vi "PalmSense Configure.vi"(8 "error in (no error)":errorcluster, 10 "Message Data":variant, 11 "Data Cluster":T1) -> (0 "error out":errorcluster, 2 "Send Resp":bool, 3 "Data Cluster out":T1)   [LabVIEW 2020, in "PalmSens.lvlib"]
uses:
  PalmSens.lvlib
  PalmSense Hardware Configuration.ctl
  <instrlib>/PalmSens SDK for LabVIEW 5.10/PalmSens/PalmSens.lvclass
  support/Message Queue/Message Cluster.ctl
  support/Message Queue/Message Queue.lvlib
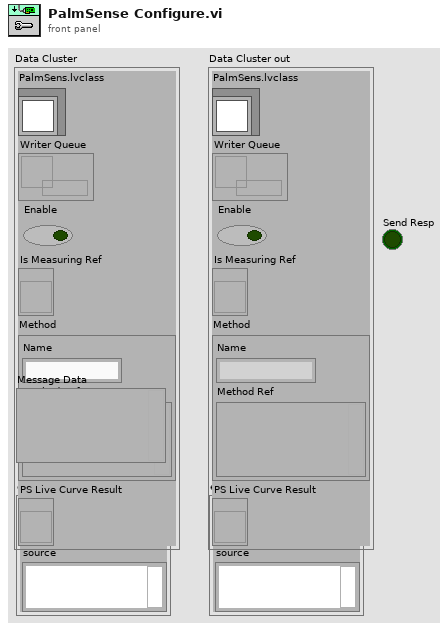
[diagram p1: front panel]
types:
  T1 = typedef "PalmSens.lvlib/PalmSense Hardware Configuration.ctl" = cluster{"PalmSens.lvclass":refnum<class "PalmSens.lvclass">, "Writer Queue":refnum<queue>, "Enable":bool, "Is Measuring Ref":refnum<vi>, "Method":cluster{"Name":string, "Method Ref":variant}, "PS Live Curve Result":refnum<vi>}
  T2 = typedef "Message Queue.lvlib/Message Cluster.ctl" = cluster{"Message":string, "Message Data":variant}
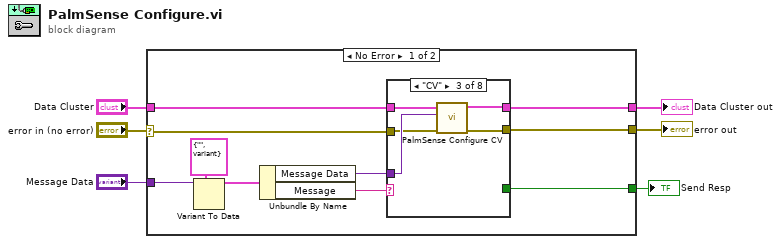
[diagram p0: block diagram]
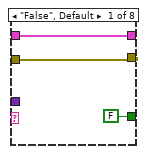
[diagram p2: hidden frame]
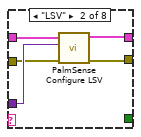
[diagram p3: hidden frame]
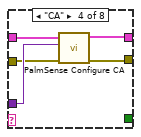
[diagram p4: hidden frame]
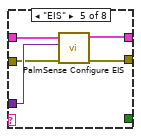
[diagram p5: hidden frame]
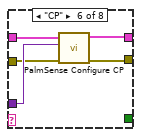
[diagram p6: hidden frame]
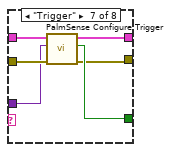
[diagram p7: hidden frame]
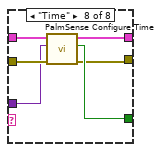
[diagram p8: hidden frame]
diagram:
  n1 = case shown="No Error" "error in (no error)" {
    selector: "error in (no error)" -> [w11 w57]
    tunnel: [w16 w57] -> w6
    tunnel: "Data Cluster" -> [w8 w58]
    tunnel: [w7 w58] -> w4
    tunnel: "Message Data" -> [w12 _]
    tunnel: [w9 _] -> w1
    frame No Error {
      n2 = Variant To Data(type=T2 {"Message"="", "Message Data"=variant} ("element"), Variant=w12) -> (data=w14:T2)  [unwired: 1 in, 1 out]
      n3 = Unbundle By Name(w14) -> ("Message Data"=w10:variant, "Message"=w15:string)
      n4 = case shown="\"CV\"" w15 {
        tunnel: w10 -> [_ w22 w27 w32 w37 w42 w45 w51]
        tunnel: [w19 w23 w28 w33 w38 w43 w49 w55] -> w7
        tunnel: w8 -> [w19 w24 w29 w34 w39 w44 w50 w56]
        tunnel: w11 -> [w18 w21 w26 w31 w36 w41 w46 w52]
        tunnel: [w18 w20 w25 w30 w35 w40 w47 w53] -> w16
        tunnel: [FALSE ("Send Resp") _ _ _ _ _ w48 w54] -> w9
        frame "False", Default {
        }
        frame "LSV" {
          n5 = call "PalmSense Configure LSV.vi"("error in (no error)"=w21, "Message Data"=w22, "Data Cluster in"=w24) -> ("error out"=w20:errorcluster, "Data Cluster out"=w23:T1)  [unwired: 7 in]
        }
        frame "CV" {
          n6 = call "PalmSense Configure CV.vi"("error in (no error)"=w26, "Message Data"=w27, "Data Cluster in"=w29) -> ("error out"=w25:errorcluster, "Data Cluster out"=w28:T1)  [unwired: 7 in]
        }
        frame "CA" {
          n7 = call "PalmSense Configure CA.vi"("error in (no error)"=w31, "Message Data"=w32, "Data Cluster in"=w34) -> ("error out"=w30:errorcluster, "Data Cluster out"=w33:T1)  [unwired: 7 in]
        }
        frame "EIS" {
          n8 = call "PalmSense Configure EIS.vi"("error in (no error)"=w36, "Message Data"=w37, "Data Cluster in"=w39) -> ("error out"=w35:errorcluster, "Data Cluster out"=w38:T1)  [unwired: 7 in]
        }
        frame "CP" {
          n9 = call "PalmSense Configure CP.vi"("error in (no error)"=w41, "Message Data"=w42, "Data Cluster in"=w44) -> ("error out"=w40:errorcluster, "Data Cluster out"=w43:T1)  [unwired: 7 in]
        }
        frame "Trigger" {
          n10 = call "PalmSense Configure Trigger.vi"("error in (no error)"=w46, "Message Data"=w45, "Data Cluster in"=w50) -> ("error out"=w47:errorcluster, "Send Resp"=w48:bool, "Data Cluster out"=w49:T1)  [unwired: 6 in]
        }
        frame "Time" {
          n11 = call "PalmSense Configure Time.vi"("error in (no error)"=w52, "Message Data"=w51, "Data Cluster in"=w56) -> ("error out"=w53:errorcluster, "Send Resp"=w54:bool, "Data Cluster out"=w55:T1)  [unwired: 6 in]
        }
      }
    }
    frame Error {
    }
  }
  "error out" <- w6
  "Data Cluster out" <- w4
  "Send Resp" <- w1
